vi "aoc-2025-d01-1.vi"() -> ()   [LabVIEW 2020]
panel:
  out "Array":i32[](array[numeric])
  out "size(s)":i32
  out "array":i32[](array[numeric])
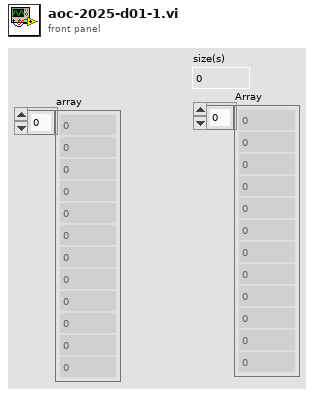
[diagram p1: front panel]
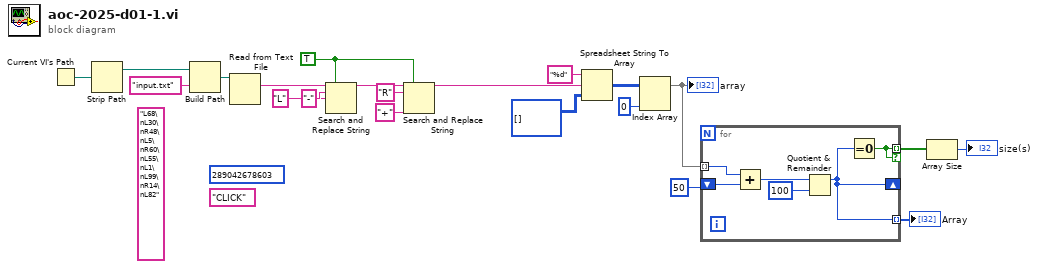
[diagram p0: block diagram]
diagram:
  (unwired) "CLICK"
  (unwired) u64 289042678603
  (unwired) "L68\nL30\nR48\nL5\nR60\nL55\nL1\nL99\nR14\nL82"
  w20 = TRUE ("replace all? (F)")
  n1 = Current VI's Path() -> (path=w5:path)
  n2 = Strip Path(path=w5) -> (stripped path=w4:path)  [unwired: 1 out]
  n3 = Build Path(base path=w4, name or relative path="input.txt") -> (appended path=w2:path)
  n4 = Read from Text File(file (use dialog)=w2) -> (text=w1:string)  [unwired: 3 in, 3 out]
  n5 = Search and Replace String(replace all?=w20, input string=w1, search string="L" ("replace string (\"\")"), replace string="-" ("replace string (\"\")")) -> (result string=w21:string)  [unwired: 4 in, 3 out]
  n6 = Search and Replace String(replace all?=w20, input string=w21, search string="R", replace string="+" ("replace string (\"\")")) -> (result string=w15:string)  [unwired: 4 in, 3 out]
  n7 = Spreadsheet String To Array(format string="%d", spreadsheet string=w15, array type (2D Dbl)=i32[][] []) -> (array=w12:i32[][])  [unwired: 1 in]
  n8 = Index Array(array=w12, index (col)=0 ("disabled index (col)")) -> (element=w10:i32[])  [unwired: 1 in]
  "array" <- w10
  n9 = for {
    tunnel: w10 -> [w27] mode=indexing
    shift-right: [w22] -> _
    shift-left: 50 -> [w26]
    tunnel: [w23] -> w8 mode=indexing if=w23
    tunnel: [w22] -> w6 mode=indexing
    n10 = Add(x=w27, y=w26) -> (x+y=w25:i32)
    n11 = Quotient & Remainder(x=w25, y=100) -> (x-y*floor(x/y)=w22:i32)  [unwired: 1 out]
    n12 = Equal To 0?(x=w22) -> (x = 0?=w23:bool)
  }
  "Array" <- w6
  n13 = Array Size(array=w8) -> (size(s)=→"size(s)":i32)
